vi "update images count.vi"(8 "error in (no error)":errorcluster, 9 "Y axis data":i32[](array[numeric]), 10 "x axis data":i32[](array[numeric]), 11 "Image in":dbl[][](array[numeric])) -> (0 "error out":errorcluster, 3 "Image Out":dbl[][](array[numeric]))   [LabVIEW 2016]
doc: "This vi takes the realtime data coming from the pixie 4 and determines which x and y\ncomponents to display. It then sorts them and them to the image to be displayed on\nthe front panel"
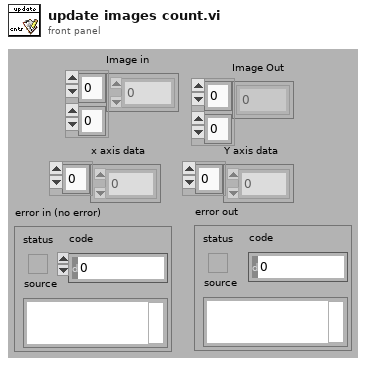
[diagram p1: front panel]
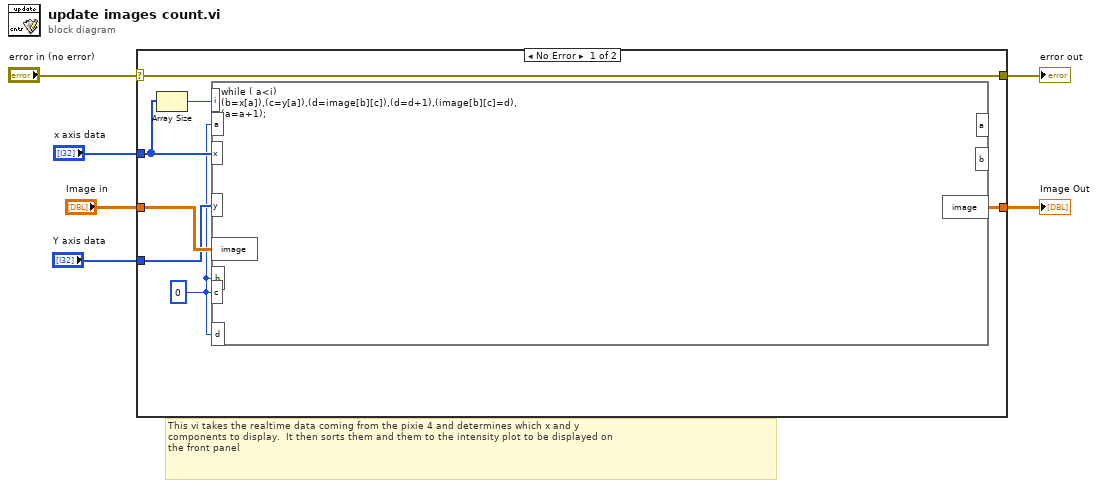
[diagram p0: block diagram]
diagram:
  # "This vi takes the realtime data coming from the pixie 4 and determines which x and y\ncomponents to display.  It then sorts them and them to the intensity plot to be displayed on\nthe front panel"
  n1 = case shown="No Error" "error in (no error)" {
    selector: "error in (no error)" -> [w13 w14]
    tunnel: "x axis data" -> [w10 _]
    tunnel: [w13 w14] -> w5
    tunnel: [w7 w15] -> w4
    tunnel: "Image in" -> [w12 w15]
    tunnel: "Y axis data" -> [w11 _]
    frame No Error {
      w8 = 0 ("input variable")
      n2 = Array Size(array=w10) -> (size(s)=w9:i32)
      n3 = formula code="while ( a<i)\n(b=x[a]),(c=y[a]),(d=image[b][c]),(d=d+1),(image[b][c]=d),\n(a=a+1);"("x"=w10, "y"=w11, "image"=w12, "i"=w9, "a"=w8, "b"=w8, "c"=w8, "d"=w8) -> ("image"=w7:dbl[][])  [unwired: 2 out]
    }
    frame Error {
    }
  }
  "error out" <- w5
  "Image Out" <- w4
